vi "SwerveDriveOutput.vi"() -> ()   [LabVIEW 2019]
doc: "This VI runs feedback and feedforward control loops, manages safety interlocks, and sends commands to the swerve drive motors."
uses:
  <vilib>/Rock Robotics/WPI/ThirdParty/Phoenix-LabVIEW/Motor Controller/Controls/CTRE_Phoenix_MotorControl_SupplyCurrentLimitConfiguration.ctl
  <vilib>/Rock Robotics/WPI/ThirdParty/Phoenix-LabVIEW/Motor Controller/Controls/CTRE_Phoenix_MotorControl_ControlMode.ctl
  <vilib>/Rock Robotics/WPI/Solenoid/WPI_SolenoidValue.ctl
  5bc46b9e-4d4b-4873-ab3e-533fd441fb60.vi
  4c0f1fb3-de9e-41af-b613-55c778746a69.vi
  refnums.vi
  outputs.vi
  dsdata.vi
  sensors.vi
  GRNF_CTREMotor.vi
  TAI_Motor.vi
  <vilib>/Rock Robotics/WPI/ThirdParty/Phoenix-LabVIEW/Motor Controller/Get/CTRE_Phoenix_MotorController_GetVoltage.vi
  <vilib>/Rock Robotics/WPI/Solenoid/WPI_SolenoidSetEnum.vi
  GRNF_GenericSolenoid.vi
  TAI_Solenoid.vi
  robotprofile.vi
panel:
  in  "Falcon PID":T1={"P Gain"=0.0001, "I Gain"=0.0, "D Gain"=0.0, "F Gain"=0.00017, "I Zone"=200.0, "Min Output"=-1.0, "Max Output"=1.0} {"Max Output" min=-1.0 max=1.0 step=0.01; "Min Output" min=-1.0 max=1.0 step=0.01; "I Zone" step=0.01; "F Gain" step=0.01; "D Gain" step=0.01; "I Gain" step=0.01; "P Gain" min=0.0 step=0.01}
  in  "Plot":u16(ring) items=["No Plot", "Wheel_0", "Wheel_1", "Wheel_2", "Wheel_3"]
  out "Drive Wheels":T2(graph)
  in  "Max Velocity (rpm)":dbl=5700.0
  in  "Min Velocity (rpm)":dbl=10.0
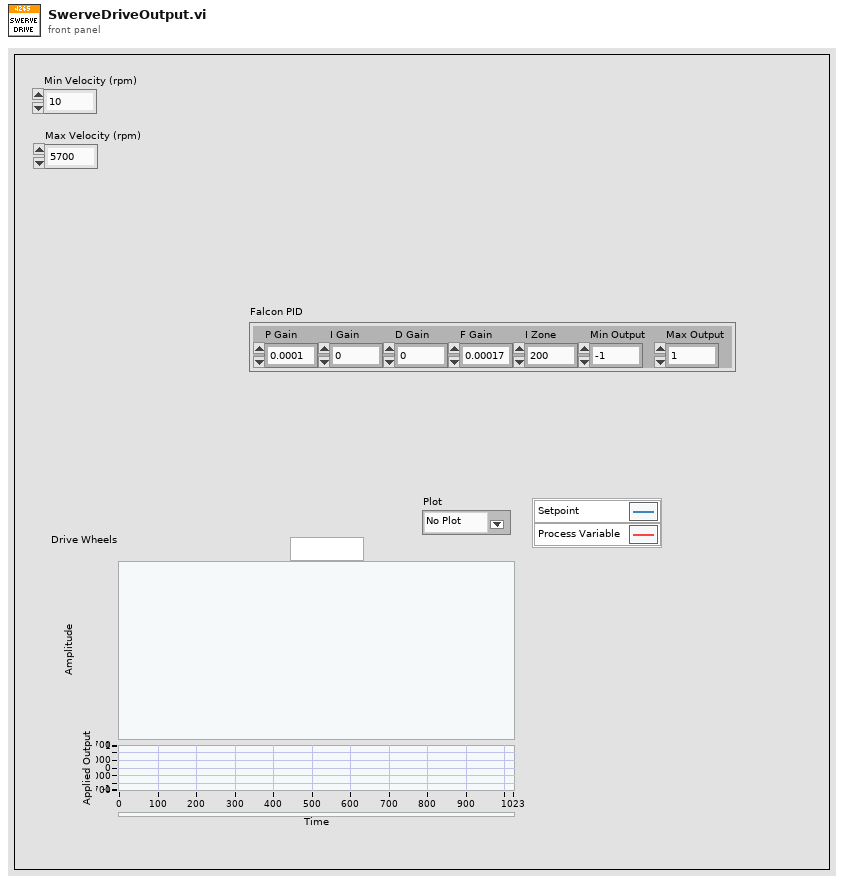
[diagram p1: front panel]
types:
  T1 = cluster{"P Gain":dbl, "I Gain":dbl, "D Gain":dbl, "F Gain":dbl, "I Zone":dbl, "Min Output":dbl, "Max Output":dbl}
  T2 = cluster{"Sensor Velocity":dbl, "Setpoint":dbl, "Applied Output":dbl}
  T3 = typedef "CTRE_Phoenix_MotorControl_ControlMode.ctl" = u16
  T4 = typedef "CTRE_Phoenix_MotorControl_SupplyCurrentLimitConfiguration.ctl" = cluster{"Enable?":bool, "Current Limit":dbl, "Threshold Current":dbl, "Threshold Time":dbl}
  T5 = cluster{"P Gain":bool, "I Gain":bool, "D Gain":bool, "F Gain":bool, "I Zone":bool, "Min Output":bool, "Max Output":bool}
  T6 = typedef "WPI_MotorControlDeviceRef.ctl" = cluster{"DeviceStatus":errorcluster, "Type":T7, "PWM":cluster{"PWM Channel":T8, "DeadBand":T9}, "CAN":cluster{"Device Number":u8, "SetOutput VI Ref":variant, "GetOutput VI Ref":variant, "Enable VI Ref":variant, "Disable VI Ref":variant, "Data":variant}, "Invert":bool, "DIO PWM":cluster{"PWM \"Enable\" Channel":T8, "DIOChannel":T10, "PWM Rate":dbl}}
  T7 = typedef "WPI_MotorControlType.ctl" = enum16{"PWM", "CAN", "DIO PWM"}
  T8 = typedef "FPGA_DIOPWMChannel.ctl" = enum8{"PWM 0", "PWM 1", "PWM 2", "PWM 3", "PWM 4", "PWM 5", "PWM 6", "PWM 7", "PWM 8", "PWM 9", "PWM MXP 0", "PWM MXP 1", "PWM MXP 2", "PWM MXP 3", "PWM MXP 4", "PWM MXP 5", "PWM MXP 6", "PWM MXP 7", "PWM MXP 8", "PWM MXP 9", "Invalid"}
  T9 = typedef "WPI_PWMDeadband.ctl" = cluster{"Name":string, "maxPositivePwm":i32, "minPositivePwm":i32, "centerPwm":i32, "maxNegativePwm":i32, "minNegativePwm":i32, "angularRange":u16}
  T10 = typedef "FPGA_DIOChannel.ctl" = enum8{"DIO 0", "DIO 1", "DIO 2", "DIO 3", "DIO 4", "DIO 5", "DIO 6", "DIO 7", "DIO 8", "DIO 9", "DIO MXP 0", "DIO MXP 1", "DIO MXP 2", "DIO MXP 3", "DIO MXP 4", "DIO MXP 5", "DIO MXP 6", "DIO MXP 7", "DIO MXP 8", "DIO MXP 9", "DIO MXP 10", "DIO MXP 11", "DIO MXP 12", "DIO MXP 13", "DIO MXP 14", "DIO MXP 15", "SPI Port CS1", "SPI Port CS2", "SPI Port CS3", "SPI Port MISO", "SPI Port MOSI", "Invalid"}
  T11 = typedef "WPI_SolenoidValue.ctl" = enum16{"Off", "On", "Forward", "Reverse"}
  T12 = typedef "WPI_SolenoidDevRef.ctl" = cluster{"DevStatus":errorcluster, "Pneumatics Control Module":u8, "Forward Solenoid Channel":T13, "Reverse Solenoid Channel":T13}
  T13 = typedef "WPI_SolenoidChannel.ctl" = enum8{"Solenoid 0", "Solenoid 1", "Solenoid 2", "Solenoid 3", "Solenoid 4", "Solenoid 5", "Solenoid 6", "Solenoid 7", "Invalid"}
  T14 = cluster{"Interlock Output":bool, "millisecond timer value":u32}
  T15 = cluster{dbl, "Swerve_0_Drive_Motor (rpm)":dbl, "Percent Output":dbl}
  T16 = cluster{dbl, "Swerve_1_Drive_Motor (rpm)":dbl, "Percent Output":dbl}
  T17 = cluster{dbl, "Swerve_2_Drive_Motor (rpm)":dbl, "Percent Output":dbl}
  T18 = cluster{dbl, "Swerve_3_Drive_Motor (rpm)":dbl, "Percent Output":dbl}
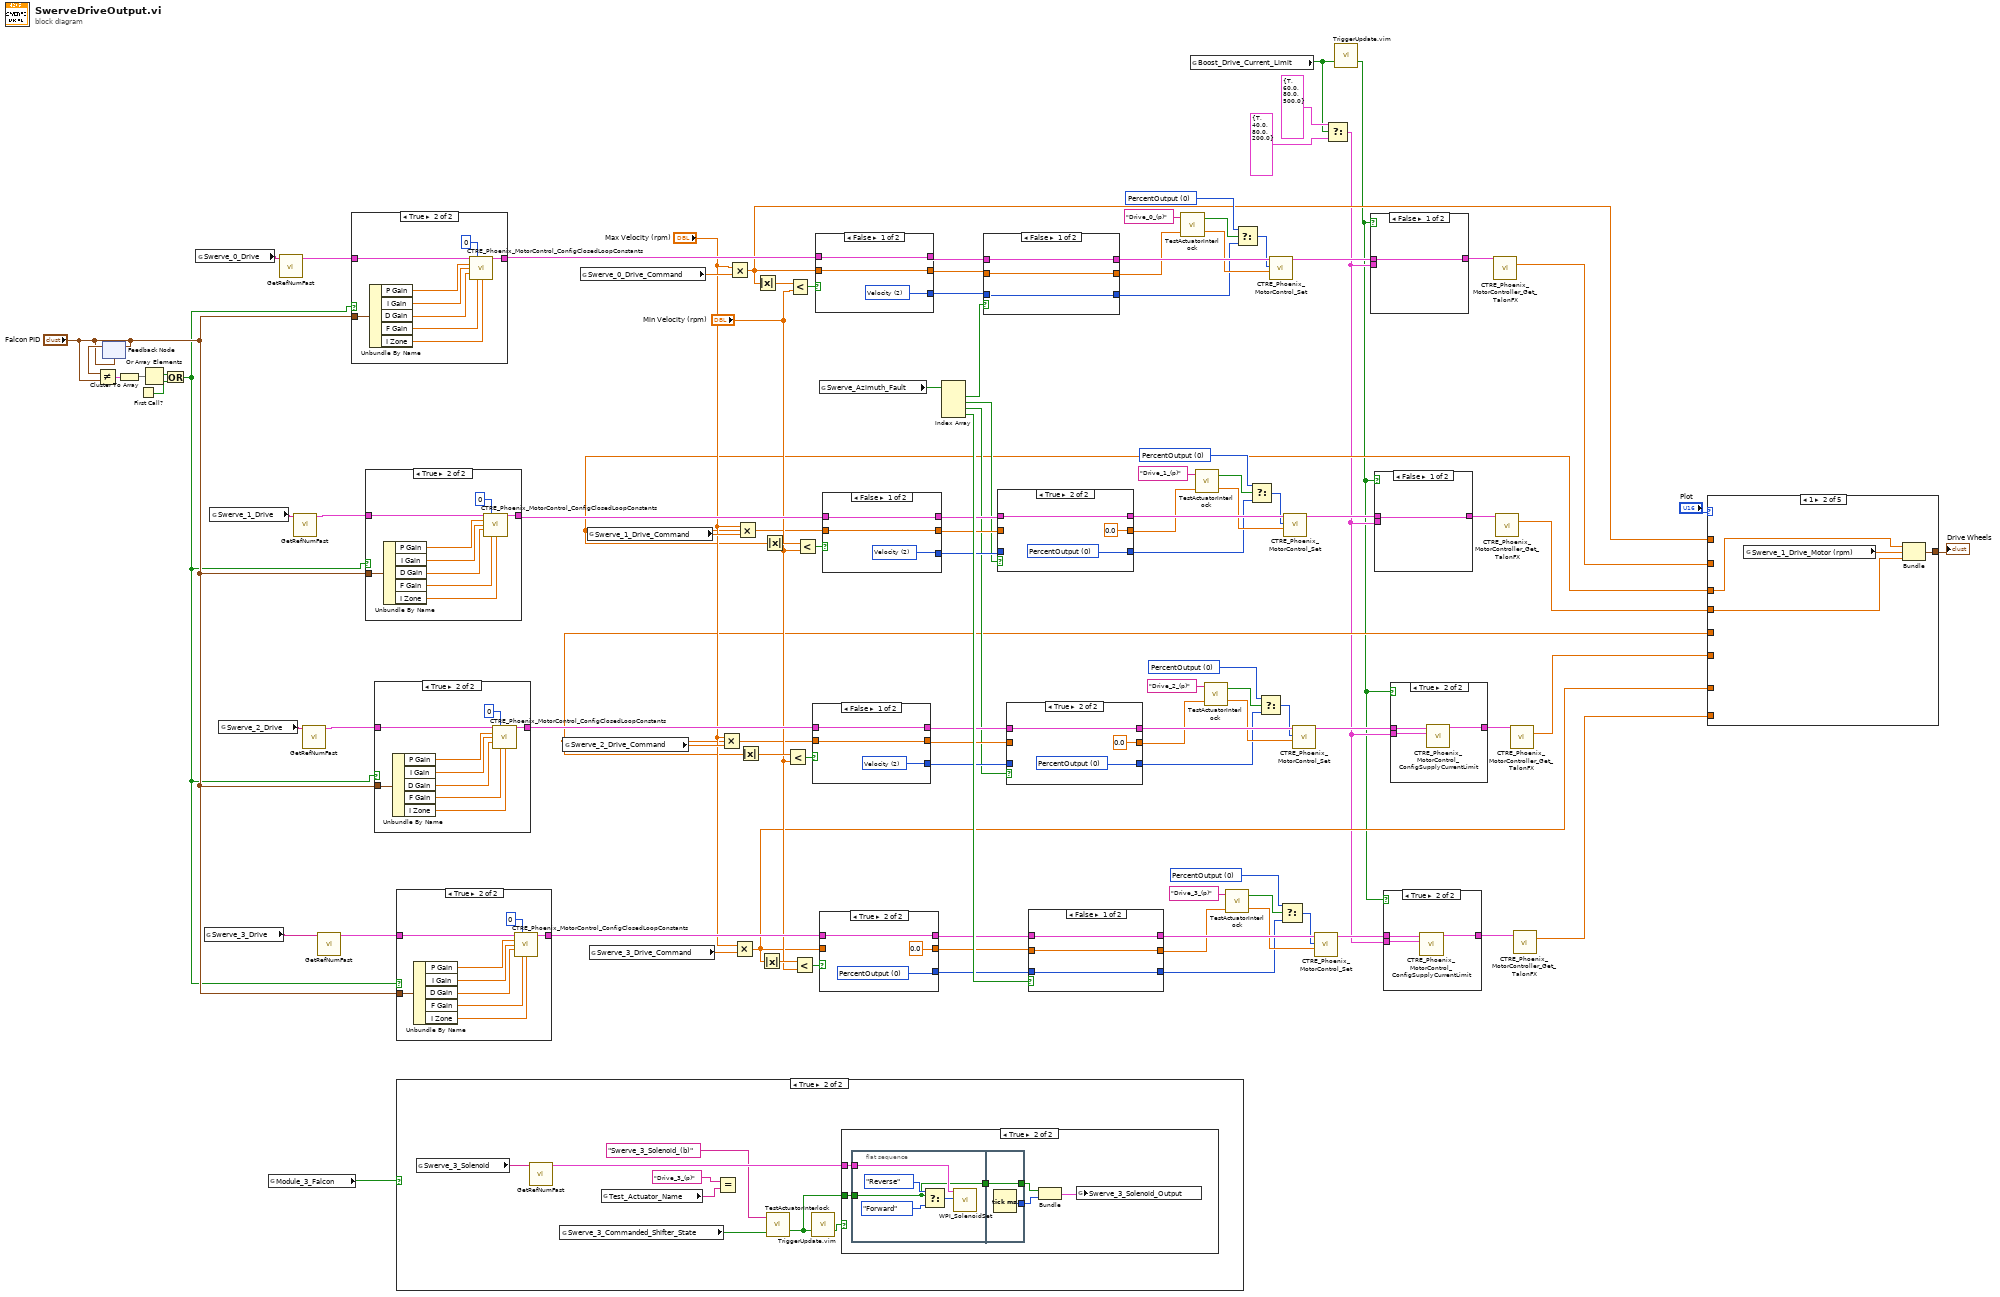
[diagram p0: block diagram]
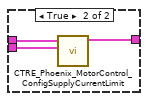
[diagram p6: hidden frame]
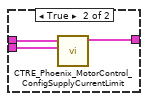
[diagram p7: hidden frame]
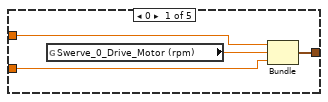
[diagram p8: hidden frame]
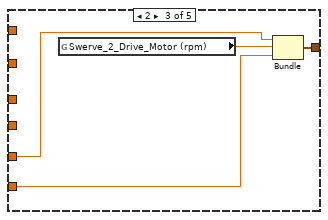
[diagram p9: hidden frame]
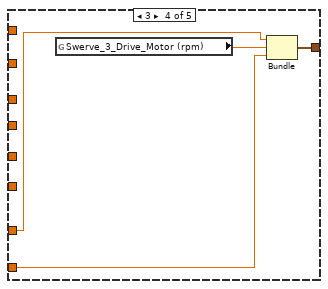
[diagram p10: hidden frame]
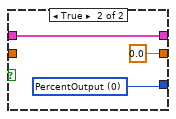
[diagram p12: hidden frame]
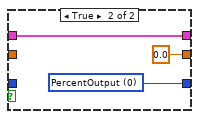
[diagram p13: hidden frame]
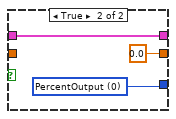
[diagram p15: hidden frame]
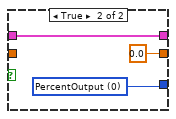
[diagram p18: hidden frame]
diagram:
  w33 = T3 0 items=["PercentOutput"=0, "Position"=1, "Velocity"=2, "Current"=3, "Follower"=5, "MotionProfile"=6, "MotionMagic"=7, "MotionProfileArc"=10, "Disabled"=15] ("Control Mode")
  w50 = T3 0 items=["PercentOutput"=0, "Position"=1, "Velocity"=2, "Current"=3, "Follower"=5, "MotionProfile"=6, "MotionMagic"=7, "MotionProfileArc"=10, "Disabled"=15] ("Control Mode")
  w67 = T3 0 items=["PercentOutput"=0, "Position"=1, "Velocity"=2, "Current"=3, "Follower"=5, "MotionProfile"=6, "MotionMagic"=7, "MotionProfileArc"=10, "Disabled"=15] ("Control Mode")
  w83 = T3 0 items=["PercentOutput"=0, "Position"=1, "Velocity"=2, "Current"=3, "Follower"=5, "MotionProfile"=6, "MotionMagic"=7, "MotionProfileArc"=10, "Disabled"=15] ("Control Mode")
  n1 = feedback #1("Falcon PID") -> (w89:T1)
  n2 = Not Equal?(x=w89, y="Falcon PID") -> (x != y?=w94:T5)
  n3 = feedback-in #1("Falcon PID") -> ()
  n4 = Cluster To Array(cluster=w94) -> (array=w95:bool[])
  n5 = First Call?() -> (First Call?: T/F=w92:bool)
  n6 = Or Array Elements(Boolean array=w95) -> (logical OR=w93:bool)
  n7 = Or(x=w93, y=w92) -> (x .or. y?=w27:bool)
  n8 = global read "refnums.vi" "Swerve_0_Drive"() -> (w45:string)
  n9 = global read "refnums.vi" "Swerve_3_Drive"() -> (w90:string)
  n10 = global read "refnums.vi" "Swerve_1_Drive"() -> (w62:string)
  n11 = global read "refnums.vi" "Swerve_2_Drive"() -> (w79:string)
  n12 = global read "robotprofile.vi" "Module_3_Falcon"() -> (w1:bool)
  n13 = call-poly "GetRefNumFast.vi"("RefNum Name"=w45) -> ("Device Reference"=w29:T6)  [unwired: 5 in, 1 out]
  n14 = call-poly "GetRefNumFast.vi"("RefNum Name"=w62) -> ("Device Reference"=w46:T6)  [unwired: 5 in, 1 out]
  n15 = call-poly "GetRefNumFast.vi"("RefNum Name"=w79) -> ("Device Reference"=w63:T6)  [unwired: 5 in, 1 out]
  n16 = call-poly "GetRefNumFast.vi"("RefNum Name"=w90) -> ("Device Reference"=w96:T6)  [unwired: 5 in, 1 out]
  n17 = case shown="True" w27 {
    tunnel: w29 -> [w107 w115]
    tunnel: "Falcon PID" -> [_ w114]
    tunnel: [w107 w116] -> w44
    frame False {
    }
    frame True {
      n18 = Unbundle By Name(w114) -> ("P Gain"=w113:dbl, "I Gain"=w112:dbl, "D Gain"=w111:dbl, "F Gain"=w110:dbl, "I Zone"=w109:dbl)
      n19 = call <vilib>:"CTRE_Phoenix_MotorControl_ConfigClosedLoopConstants.vi"("PhoenixMotorControlDevRef"=w115, "slotIdx"=0, "P"=w113, "I"=w112, "D"=w111, "F"=w110, "I Zone"=w109) -> ("PhoenixMotorControlDevRef"=w116:T6)  [unwired: 7 in, 1 out]
    }
  }
  n20 = case shown="True" w27 {
    tunnel: w46 -> [w117 w125]
    tunnel: "Falcon PID" -> [_ w124]
    tunnel: [w117 w126] -> w61
    frame False {
    }
    frame True {
      n21 = Unbundle By Name(w124) -> ("P Gain"=w118:dbl, "I Gain"=w123:dbl, "D Gain"=w122:dbl, "F Gain"=w121:dbl, "I Zone"=w120:dbl)
      n22 = call <vilib>:"CTRE_Phoenix_MotorControl_ConfigClosedLoopConstants.vi"("PhoenixMotorControlDevRef"=w125, "slotIdx"=0, "P"=w118, "I"=w123, "D"=w122, "F"=w121, "I Zone"=w120) -> ("PhoenixMotorControlDevRef"=w126:T6)  [unwired: 7 in, 1 out]
    }
  }
  n23 = case shown="True" w27 {
    tunnel: w63 -> [w127 w135]
    tunnel: "Falcon PID" -> [_ w134]
    tunnel: [w127 w136] -> w78
    frame False {
    }
    frame True {
      n24 = Unbundle By Name(w134) -> ("P Gain"=w133:dbl, "I Gain"=w132:dbl, "D Gain"=w131:dbl, "F Gain"=w130:dbl, "I Zone"=w129:dbl)
      n25 = call <vilib>:"CTRE_Phoenix_MotorControl_ConfigClosedLoopConstants.vi"("PhoenixMotorControlDevRef"=w135, "slotIdx"=0, "P"=w133, "I"=w132, "D"=w131, "F"=w130, "I Zone"=w129) -> ("PhoenixMotorControlDevRef"=w136:T6)  [unwired: 7 in, 1 out]
    }
  }
  n26 = case shown="True" w27 {
    tunnel: w96 -> [w137 w145]
    tunnel: "Falcon PID" -> [_ w144]
    tunnel: [w137 w146] -> w101
    frame False {
    }
    frame True {
      n27 = Unbundle By Name(w144) -> ("P Gain"=w143:dbl, "I Gain"=w142:dbl, "D Gain"=w141:dbl, "F Gain"=w140:dbl, "I Zone"=w139:dbl)
      n28 = call <vilib>:"CTRE_Phoenix_MotorControl_ConfigClosedLoopConstants.vi"("PhoenixMotorControlDevRef"=w145, "slotIdx"=0, "P"=w143, "I"=w142, "D"=w141, "F"=w140, "I Zone"=w139) -> ("PhoenixMotorControlDevRef"=w146:T6)  [unwired: 7 in, 1 out]
    }
  }
  n29 = case shown="True" w1 {
    frame False {
    }
    frame True {
      n30 = global read "refnums.vi" "Swerve_3_Solenoid"() -> (w150:string)
      n31 = call-poly "GetRefNumFast.vi"("RefNum Name"=w150) -> ("Device Reference"=w152:T12)  [unwired: 5 in, 1 out]
      n32 = global read "outputs.vi" "Swerve_3_Commanded_Shifter_State"() -> (w149:bool)
      n33 = global read "dsdata.vi" "Test_Actuator_Name"() -> (w147:string)
      n34 = Equal?(x="Drive_3_(p)" ("Actuator_Name"), y=w147) -> ()  [unwired: 1 out]
      n35 = call-poly "TestActuatorInterlock.vi"("Normal Output"=w149, "Actuator Name"="Swerve_3_Solenoid_(b)" ("Actuator_Name")) -> ("Interlock Output"=w153:bool)  [unwired: 1 in, 1 out]
      n36 = call "TriggerUpdate.vim"("Trigger"=w153) -> ("Update"=w154:bool)  [unwired: 2 in]
      n37 = case shown="True" w154 {
        tunnel: w152 -> [_ w160]
        tunnel: w153 -> [_ w159]
        frame False {
        }
        frame True {
          n38 = flat-sequence {
            tunnel: w160 -> [w162]
            tunnel: w159 -> [w161]
            tunnel: [w161] -> w158
            tunnel: w158 -> [w167]
            tunnel: [w167] -> w156
            tunnel: [w166] -> w155
            frame #0 {
              n39 = Select(t=WPI_SolenoidValue."Reverse" ("Value"), s=w161, f=WPI_SolenoidValue."Forward" ("Value")) -> (s? t:f=w163:T11)
              n40 = call-poly <vilib>:"WPI_SolenoidSet.vi"("Value"=w163, "SolenoidDevRef"=w162) -> ()  [unwired: 8 in, 2 out]
            }
            frame #1 {
              n41 = Tick Count (ms)() -> (millisecond timer value=w166:u32)
            }
          }
          n42 = Bundle("Interlock Output"=w156, "millisecond timer value"=w155) -> (w157:T14)  [unwired: 1 in]
          n43 = global write "outputs.vi" "Swerve_3_Solenoid_Output"(w157) -> ()
        }
      }
    }
  }
  n44 = global read "outputs.vi" "Swerve_2_Drive_Command"() -> (w64:dbl)
  n45 = global read "outputs.vi" "Swerve_0_Drive_Command"() -> (w30:dbl)
  n46 = global read "outputs.vi" "Swerve_1_Drive_Command"() -> (w47:dbl)
  n47 = global read "outputs.vi" "Swerve_3_Drive_Command"() -> (w80:dbl)
  n48 = Multiply(x="Max Velocity (rpm)", y=w64) -> (x*y=w13:dbl)
  n49 = Multiply(x="Max Velocity (rpm)", y=w30) -> (x*y=w16:dbl)
  n50 = Multiply(x="Max Velocity (rpm)", y=w80) -> (x*y=w12:dbl)
  n51 = Multiply(x="Max Velocity (rpm)", y=w47) -> (x*y=w14:dbl)
  n52 = Absolute Value(x=w13) -> (abs(x)=w73:dbl)
  n53 = Absolute Value(x=w16) -> (abs(x)=w39:dbl)
  n54 = Absolute Value(x=w12) -> (abs(x)=w91:dbl)
  n55 = Absolute Value(x=w14) -> (abs(x)=w56:dbl)
  n56 = Less?(x=w73, y="Min Velocity (rpm)") -> (x < y?=w77:bool)
  n57 = Less?(x=w39, y="Min Velocity (rpm)") -> (x < y?=w43:bool)
  n58 = Less?(x=w91, y="Min Velocity (rpm)") -> (x < y?=w100:bool)
  n59 = Less?(x=w56, y="Min Velocity (rpm)") -> (x < y?=w60:bool)
  n60 = case shown="False" w77 {
    tunnel: [w170 w173] -> w74
    tunnel: w78 -> [w170 w173]
    tunnel: [w169 0.0 ("Command")] -> w75
    tunnel: w13 -> [w169 _]
    tunnel: [w168 w171] -> w76
    frame False {
      w168 = T3 2 items=["PercentOutput"=0, "Position"=1, "Velocity"=2, "Current"=3, "Follower"=5, "MotionProfile"=6, "MotionMagic"=7, "MotionProfileArc"=10, "Disabled"=15] ("Control Mode")
    }
    frame True {
      w171 = T3 0 items=["PercentOutput"=0, "Position"=1, "Velocity"=2, "Current"=3, "Follower"=5, "MotionProfile"=6, "MotionMagic"=7, "MotionProfileArc"=10, "Disabled"=15] ("Control Mode")
    }
  }
  n61 = case shown="False" w43 {
    tunnel: [w176 w179] -> w40
    tunnel: w44 -> [w176 w179]
    tunnel: [w175 0.0 ("Command")] -> w41
    tunnel: w16 -> [w175 _]
    tunnel: [w174 w177] -> w42
    frame False {
      w174 = T3 2 items=["PercentOutput"=0, "Position"=1, "Velocity"=2, "Current"=3, "Follower"=5, "MotionProfile"=6, "MotionMagic"=7, "MotionProfileArc"=10, "Disabled"=15] ("Control Mode")
    }
    frame True {
      w177 = T3 0 items=["PercentOutput"=0, "Position"=1, "Velocity"=2, "Current"=3, "Follower"=5, "MotionProfile"=6, "MotionMagic"=7, "MotionProfileArc"=10, "Disabled"=15] ("Control Mode")
    }
  }
  n62 = global read "sensors.vi" "Swerve_Azimuth_Fault"() -> (w106:bool[])
  n63 = case shown="True" w100 {
    tunnel: [w182 w185] -> w97
    tunnel: w101 -> [w182 w185]
    tunnel: [w181 0.0 ("Command")] -> w98
    tunnel: w12 -> [w181 _]
    tunnel: [w180 w183] -> w99
    frame False {
      w180 = T3 2 items=["PercentOutput"=0, "Position"=1, "Velocity"=2, "Current"=3, "Follower"=5, "MotionProfile"=6, "MotionMagic"=7, "MotionProfileArc"=10, "Disabled"=15] ("Control Mode")
    }
    frame True {
      w183 = T3 0 items=["PercentOutput"=0, "Position"=1, "Velocity"=2, "Current"=3, "Follower"=5, "MotionProfile"=6, "MotionMagic"=7, "MotionProfileArc"=10, "Disabled"=15] ("Control Mode")
    }
  }
  n64 = case shown="False" w60 {
    tunnel: [w188 w191] -> w57
    tunnel: w61 -> [w188 w191]
    tunnel: [w187 0.0 ("Command")] -> w58
    tunnel: w14 -> [w187 _]
    tunnel: [w186 w189] -> w59
    frame False {
      w186 = T3 2 items=["PercentOutput"=0, "Position"=1, "Velocity"=2, "Current"=3, "Follower"=5, "MotionProfile"=6, "MotionMagic"=7, "MotionProfileArc"=10, "Disabled"=15] ("Control Mode")
    }
    frame True {
      w189 = T3 0 items=["PercentOutput"=0, "Position"=1, "Velocity"=2, "Current"=3, "Follower"=5, "MotionProfile"=6, "MotionMagic"=7, "MotionProfileArc"=10, "Disabled"=15] ("Control Mode")
    }
  }
  n65 = Index Array(array=w106) -> (element #1=w24:bool, element #2=w23:bool, element #3=w22:bool, element #4=w105:bool)  [unwired: 4 in]
  n66 = case shown="False" w24 {
    tunnel: [w194 w197] -> w38
    tunnel: w40 -> [w194 w197]
    tunnel: [w193 0.0 ("Command")] -> w35
    tunnel: w41 -> [w193 _]
    tunnel: w42 -> [w192 _]
    tunnel: [w192 w195] -> w32
    frame False {
    }
    frame True {
      w195 = T3 0 items=["PercentOutput"=0, "Position"=1, "Velocity"=2, "Current"=3, "Follower"=5, "MotionProfile"=6, "MotionMagic"=7, "MotionProfileArc"=10, "Disabled"=15] ("Control Mode")
    }
  }
  n67 = case shown="True" w23 {
    tunnel: [w200 w203] -> w55
    tunnel: w57 -> [w200 w203]
    tunnel: [w199 0.0 ("Command")] -> w52
    tunnel: w58 -> [w199 _]
    tunnel: w59 -> [w198 _]
    tunnel: [w198 w201] -> w49
    frame False {
    }
    frame True {
      w201 = T3 0 items=["PercentOutput"=0, "Position"=1, "Velocity"=2, "Current"=3, "Follower"=5, "MotionProfile"=6, "MotionMagic"=7, "MotionProfileArc"=10, "Disabled"=15] ("Control Mode")
    }
  }
  n68 = case shown="True" w22 {
    tunnel: [w206 w209] -> w72
    tunnel: w74 -> [w206 w209]
    tunnel: [w205 0.0 ("Command")] -> w69
    tunnel: w75 -> [w205 _]
    tunnel: w76 -> [w204 _]
    tunnel: [w204 w207] -> w66
    frame False {
    }
    frame True {
      w207 = T3 0 items=["PercentOutput"=0, "Position"=1, "Velocity"=2, "Current"=3, "Follower"=5, "MotionProfile"=6, "MotionMagic"=7, "MotionProfileArc"=10, "Disabled"=15] ("Control Mode")
    }
  }
  n69 = case shown="False" w105 {
    tunnel: [w212 w215] -> w88
    tunnel: w97 -> [w212 w215]
    tunnel: [w211 0.0 ("Command")] -> w85
    tunnel: w98 -> [w211 _]
    tunnel: w99 -> [w210 _]
    tunnel: [w210 w213] -> w82
    frame False {
    }
    frame True {
      w213 = T3 0 items=["PercentOutput"=0, "Position"=1, "Velocity"=2, "Current"=3, "Follower"=5, "MotionProfile"=6, "MotionMagic"=7, "MotionProfileArc"=10, "Disabled"=15] ("Control Mode")
    }
  }
  n70 = call-poly "TestActuatorInterlock.vi"("Normal Output"=w35, "Actuator Name"="Drive_0_(p)" ("Actuator_Name")) -> ("Interlock Output"=w34:dbl, "Testing This Actuator"=w37:bool)  [unwired: 1 in]
  n71 = global read "outputs.vi" "Boost_Drive_Current_Limit"() -> (w103:bool)
  n72 = call-poly "TestActuatorInterlock.vi"("Normal Output"=w52, "Actuator Name"="Drive_1_(p)" ("Actuator_Name")) -> ("Interlock Output"=w51:dbl, "Testing This Actuator"=w54:bool)  [unwired: 1 in]
  n73 = call-poly "TestActuatorInterlock.vi"("Normal Output"=w69, "Actuator Name"="Drive_2_(p)" ("Actuator_Name")) -> ("Interlock Output"=w68:dbl, "Testing This Actuator"=w71:bool)  [unwired: 1 in]
  n74 = call-poly "TestActuatorInterlock.vi"("Normal Output"=w85, "Actuator Name"="Drive_3_(p)" ("Actuator_Name")) -> ("Interlock Output"=w84:dbl, "Testing This Actuator"=w87:bool)  [unwired: 1 in]
  n75 = Select(t=w33, s=w37, f=w32) -> (s? t:f=w31:T3)
  n76 = Select(t=w50, s=w54, f=w49) -> (s? t:f=w48:T3)
  n77 = Select(t=w67, s=w71, f=w66) -> (s? t:f=w65:T3)
  n78 = call <vilib>:"CTRE_Phoenix_MotorControl_Set.vi"("Output"=w34, "Control Mode"=w31, "PhoenixMotorControlDevRef"=w38) -> ("PhoenixMotorControlDevRef"=w11:T6)  [unwired: 7 in, 1 out]
  n79 = Select(t=w83, s=w87, f=w82) -> (s? t:f=w81:T3)
  n80 = call <vilib>:"CTRE_Phoenix_MotorControl_Set.vi"("Output"=w51, "Control Mode"=w48, "PhoenixMotorControlDevRef"=w55) -> ("PhoenixMotorControlDevRef"=w9:T6)  [unwired: 7 in, 1 out]
  n81 = call <vilib>:"CTRE_Phoenix_MotorControl_Set.vi"("Output"=w68, "Control Mode"=w65, "PhoenixMotorControlDevRef"=w72) -> ("PhoenixMotorControlDevRef"=w7:T6)  [unwired: 7 in, 1 out]
  n82 = call <vilib>:"CTRE_Phoenix_MotorControl_Set.vi"("Output"=w84, "Control Mode"=w81, "PhoenixMotorControlDevRef"=w88) -> ("PhoenixMotorControlDevRef"=w5:T6)  [unwired: 7 in, 1 out]
  n83 = Select(t=T4 {"Enable?"=TRUE, "Current Limit"=60.0, "Threshold Current"=80.0, "Threshold Time"=500.0} ("Supply Current Limit Configuration"), s=w103, f=T4 {"Enable?"=TRUE, "Current Limit"=40.0, "Threshold Current"=80.0, "Threshold Time"=200.0} ("Supply Current Limit Configuration")) -> (s? t:f=w3:T4)
  n84 = call "TriggerUpdate.vim"("Trigger"=w103) -> ("Update"=w2:bool)  [unwired: 2 in]
  n85 = case shown="False" w2 {
    tunnel: w11 -> [w216 w219]
    tunnel: [w216 w218] -> w10
    tunnel: w3 -> [_ w217]
    frame False {
    }
    frame True {
      n86 = call <vilib>:"CTRE_Phoenix_MotorControl_ConfigSupplyCurrentLimit.vi"("Supply Current Limit Configuration"=w217, "PhoenixMotorControlDevRef"=w219) -> ("PhoenixMotorControlDevRef"=w218:T6)  [unwired: 8 in, 1 out]
    }
  }
  n87 = case shown="False" w2 {
    tunnel: w9 -> [w220 w223]
    tunnel: [w220 w222] -> w8
    tunnel: w3 -> [_ w221]
    frame False {
    }
    frame True {
      n88 = call <vilib>:"CTRE_Phoenix_MotorControl_ConfigSupplyCurrentLimit.vi"("Supply Current Limit Configuration"=w221, "PhoenixMotorControlDevRef"=w223) -> ("PhoenixMotorControlDevRef"=w222:T6)  [unwired: 8 in, 1 out]
    }
  }
  n89 = case shown="True" w2 {
    tunnel: w5 -> [w224 w227]
    tunnel: [w224 w226] -> w4
    tunnel: w3 -> [_ w225]
    frame False {
    }
    frame True {
      n90 = call <vilib>:"CTRE_Phoenix_MotorControl_ConfigSupplyCurrentLimit.vi"("Supply Current Limit Configuration"=w225, "PhoenixMotorControlDevRef"=w227) -> ("PhoenixMotorControlDevRef"=w226:T6)  [unwired: 8 in, 1 out]
    }
  }
  n91 = case shown="True" w2 {
    tunnel: w7 -> [w228 w231]
    tunnel: [w228 w230] -> w6
    tunnel: w3 -> [_ w229]
    frame False {
    }
    frame True {
      n92 = call <vilib>:"CTRE_Phoenix_MotorControl_ConfigSupplyCurrentLimit.vi"("Supply Current Limit Configuration"=w229, "PhoenixMotorControlDevRef"=w231) -> ("PhoenixMotorControlDevRef"=w230:T6)  [unwired: 8 in, 1 out]
    }
  }
  n93 = call-poly <vilib>:"CTRE_Phoenix_MotorController_Get_TalonFX.vi"("PhoenixMotorControlDevRef"=w10) -> ("Percent Output"=w20:dbl)  [unwired: 10 in, 4 out]
  n94 = call-poly <vilib>:"CTRE_Phoenix_MotorController_Get_TalonFX.vi"("PhoenixMotorControlDevRef"=w8) -> ("Percent Output"=w19:dbl)  [unwired: 10 in, 4 out]
  n95 = call-poly <vilib>:"CTRE_Phoenix_MotorController_Get_TalonFX.vi"("PhoenixMotorControlDevRef"=w6) -> ("Percent Output"=w18:dbl)  [unwired: 10 in, 4 out]
  n96 = call-poly <vilib>:"CTRE_Phoenix_MotorController_Get_TalonFX.vi"("PhoenixMotorControlDevRef"=w4) -> ("Percent Output"=w17:dbl)  [unwired: 10 in, 4 out]
  n97 = case shown="1" "Plot" {
    tunnel: [w232 w236 w240 w244 _] -> w15
    tunnel: w20 -> [w234 _ _ _ _]
    tunnel: w19 -> [_ w237 _ _ _]
    tunnel: w18 -> [_ _ w241 _ _]
    tunnel: w17 -> [_ _ _ w245 _]
    tunnel: w16 -> [w233 _ _ _ _]
    tunnel: w14 -> [_ w238 _ _ _]
    tunnel: w13 -> [_ _ w242 _ _]
    tunnel: w12 -> [_ _ _ w246 _]
    frame 0 {
      n98 = global read "sensors.vi" "Swerve_0_Drive_Motor (rpm)"() -> (w235:dbl)
      n99 = Bundle(w233, "Swerve_0_Drive_Motor (rpm)"=w235, "Percent Output"=w234) -> (w232:T15)  [unwired: 1 in]
    }
    frame 1 {
      n100 = global read "sensors.vi" "Swerve_1_Drive_Motor (rpm)"() -> (w239:dbl)
      n101 = Bundle(w238, "Swerve_1_Drive_Motor (rpm)"=w239, "Percent Output"=w237) -> (w236:T16)  [unwired: 1 in]
    }
    frame 2 {
      n102 = global read "sensors.vi" "Swerve_2_Drive_Motor (rpm)"() -> (w243:dbl)
      n103 = Bundle(w242, "Swerve_2_Drive_Motor (rpm)"=w243, "Percent Output"=w241) -> (w240:T17)  [unwired: 1 in]
    }
    frame 3 {
      n104 = global read "sensors.vi" "Swerve_3_Drive_Motor (rpm)"() -> (w247:dbl)
      n105 = Bundle(w246, "Swerve_3_Drive_Motor (rpm)"=w247, "Percent Output"=w245) -> (w244:T18)  [unwired: 1 in]
    }
    frame 4, Default {
    }
  }
  "Drive Wheels" <- w15
